vi "Fetch Measurement.vi"   [LabVIEW 2010, in "Agilent 3458.lvlib"]
doc: "Supports different methods of retrieving data from the output buffer."
uses:
  <instrlib>/Agilent 3458/Agilent 3458.lvlib
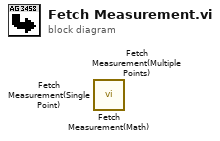
[diagram p0: block diagram]
diagram:
  n1 = call <instrlib>:"Fetch Measurement(Math).vi"() -> ()  [unwired: 9 in, 7 out]
  n2 = call <instrlib>:"Fetch Measurement(Multiple Points).vi"() -> ()  [unwired: 13 in, 3 out]
  n3 = call <instrlib>:"Fetch Measurement(Single Point).vi"() -> ()  [unwired: 13 in, 3 out]
